vi "Potenze(SubVI).vi"(8 "ultimo trigger":i32, 9 "1 trigger":i32, 10 "2":dbl[](array[numeric]), 11 "1":dbl[](array[numeric])) -> (1 "Q P.Reattiva":dbl=4.945576802306794 format="%.9f", 2 "S P.Apparente":dbl=4.945576845195044 format="%.9f", 3 "P attiva":dbl=-0.000651317328266863 format="%.9f", 4 "Rms Ch 1":dbl=-0.000651317328266863 format="%.9f", 6 "Rms Ch 2":dbl=-0.000651317328266863 format="%.9f")   [LabVIEW 2018]
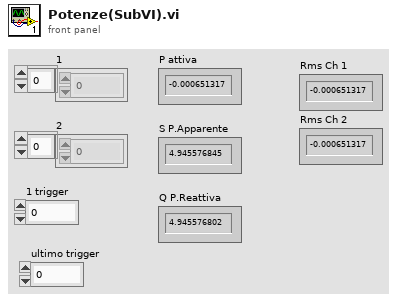
[diagram p1: front panel]
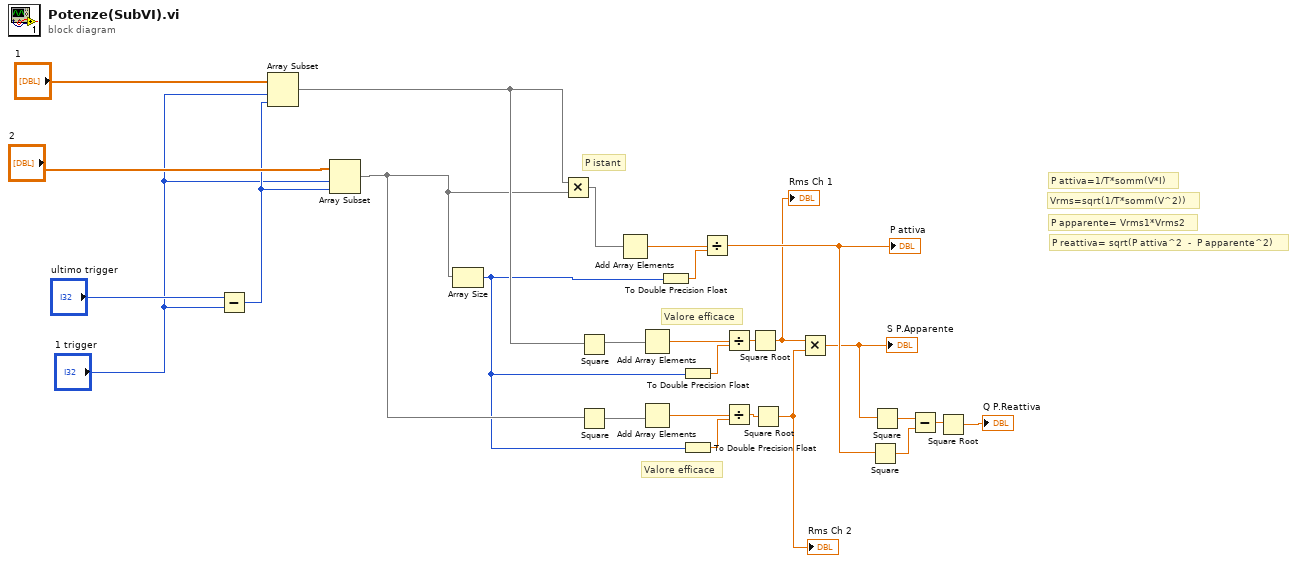
[diagram p0: block diagram]
diagram:
  # "P reattiva= sqrt(P attiva^2  -  P apparente^2)"
  # "Vrms=sqrt(1/T*somm(V^2))"
  # "P apparente= Vrms1*Vrms2"
  # "P attiva=1/T*somm(V*I)"
  # "Valore efficace"
  # "Valore efficace"
  # "P istant"
  n1 = Subtract(x="ultimo trigger", y="1 trigger") -> (x-y=w10:i32)
  n2 = Array Subset(array="1", index="1 trigger", length=w10) -> (w7:dbl[])
  n3 = Array Subset(array="2", index="1 trigger", length=w10) -> (w5:dbl[])
  n4 = Array Size(array=w5) -> (size(s)=w3:i32)
  n5 = Multiply(x=w7, y=w5) -> (x*y=w8:dbl[])
  n6 = Square(x=w7) -> (x^2=w6:dbl[])
  n7 = Square(x=w5) -> (x^2=w4:dbl[])
  n8 = Add Array Elements(numeric array=w8) -> (sum=w14:dbl)
  n9 = Add Array Elements(numeric array=w6) -> (sum=w16:dbl)
  n10 = Add Array Elements(numeric array=w4) -> (sum=w19:dbl)
  n11 = To Double Precision Float(number=w3) -> (double precision float=w15:dbl)
  n12 = To Double Precision Float(number=w3) -> (double precision float=w18:dbl)
  n13 = To Double Precision Float(number=w3) -> (double precision float=w20:dbl)
  n14 = Divide(x=w14, y=w15) -> (x/y=w23:dbl)
  "P attiva" <- w23
  n15 = Divide(x=w16, y=w18) -> (x/y=w17:dbl)
  n16 = Divide(x=w19, y=w20) -> (x/y=w21:dbl)
  n17 = Square Root(x=w17) -> (sqrt(x)=w2:dbl)
  "Rms Ch 1" <- w2
  n18 = Square Root(x=w21) -> (sqrt(x)=w1:dbl)
  "Rms Ch 2" <- w1
  n19 = Multiply(x=w2, y=w1) -> (x*y=w22:dbl)
  "S P.Apparente" <- w22
  n20 = Square(x=w23) -> (x^2=w25:dbl)
  n21 = Square(x=w22) -> (x^2=w24:dbl)
  n22 = Subtract(x=w24, y=w25) -> (x-y=w26:dbl)
  n23 = Square Root(x=w26) -> (sqrt(x)=→"Q P.Reattiva":dbl)
